vi "example.vi"   [LabVIEW 2017]
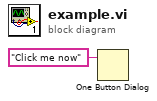
[diagram p0: block diagram]
diagram:
  n1 = One Button Dialog(message="Click me now") -> ()  [unwired: 1 in, 1 out]
